vi "viewerMain.vi"(1 "viewer.lvclass":refnum<class "viewer.lvclass">) -> (0 "viewer.lvclass 2":refnum<class "viewer.lvclass">)   [LabVIEW 2011, in "viewer.lvclass"]
uses:
  Pollers/ttm_poller_panel_class/viewer.lvclass
  viewerDataVectors.ctl
  protocols/protocol_Generic/Protocol_Generic.lvclass
  viewerSingleGraph.ctl
panel:
  out "protocol Runner error":errorcluster
  in  "ttmServer vi":path=path "D:/workspace/lumikki-devices/ttm/protocols/run_protocols/main.vi"
  in  "Updade frequency [ms]":u32=1000
  in  "Scales":T1={"Scale time"=1.0, "Scale analog displacement"=1.0, "Scale force"=1.0, "Scale digital displacement"=1.0, "Scale external"=1.0}
  in  "Tab Control":T2(tab)=enum."Force-displacement"
  in  "Front panel name":u16(ring) items=["select front panel", "Run_protocols.lvclass:main.vi"]
  out "Force-displacement":cluster{"Y":dbl[], "Y":dbl[]}[](graph)=[{"Y"=[0.5311861979208834, 0.5311861979208834, 0.6668696350036979, 0.7379313711099627, 0.8016199408837772, 0.8572989891886034, 0.9044121893788258, 0.9424888019316975, 0.9711483779210446, 0.9901045603371778, 0.999167945271476, 0.9982479743776325, 0.9873538397007164, 0.9665943918332975, 0.9361770523163061, 0.89640574115156, 0.8476778401335698, 0.7904802223420048, 0.7253843874668195, 0.6530407515722648, 0.5741721483545726, 0.4895666068265995, 0.4000694775924195, 0.30657498638352293, 0.21001729925089915, 0.11136118868665001, 0.011592393936158275, -0.0882922281826076, -0.18729466354290317, -0.28442571253646254, -0.3787148738289976], "Y"=[0.36472117505578305, 0.36472117505578305, 0.46768216950310704, 0.5255260682597803, 0.5810351605373051, 0.6339628306183481, 0.684073931524491, 0.7311458297268958, 0.7749693942622354, 0.8153499258594433, 0.852108021949363, 0.8850803737142298, 0.9141204916358583, 0.9390993563190676, 0.9599059916988695, 0.9764479580847747, 0.9886517628517197, 0.9964631869529988, 0.9998475258045683, 0.998789743470524, 0.9932945394647364, 0.9833863278718569, 0.9691091288804563, 0.9505263732101938, 0.9277206203019036, 0.9007931915226273, 0.8698637200151869, 0.8350696191922243, 0.7965654722360865, 0.7545223453168781, 0.7091270275799205]}]
  out "X-time":cluster{"Y":dbl[], "Y":dbl[]}[](graph)=[{"Y"=[56.0, 56.0, 73.0, 83.0, 93.0, 103.0, 113.0, 123.0, 133.0, 143.0, 153.0, 163.0, 173.0, 183.0, 193.0, 203.0, 213.0, 223.0, 233.0, 243.0, 253.0, 263.0, 273.0, 283.0, 293.0, 303.0, 313.0, 323.0, 333.0, 343.0, 353.0], "Y"=[0.5311861979208834, 0.5311861979208834, 0.6668696350036979, 0.7379313711099627, 0.8016199408837772, 0.8572989891886034, 0.9044121893788258, 0.9424888019316975, 0.9711483779210446, 0.9901045603371778, 0.999167945271476, 0.9982479743776325, 0.9873538397007164, 0.9665943918332975, 0.9361770523163061, 0.89640574115156, 0.8476778401335698, 0.7904802223420048, 0.7253843874668195, 0.6530407515722648, 0.5741721483545726, 0.4895666068265995, 0.4000694775924195, 0.30657498638352293, 0.21001729925089915, 0.11136118868665001, 0.011592393936158275, -0.0882922281826076, -0.18729466354290317, -0.28442571253646254, -0.3787148738289976]}, {"Y"=[56.0, 56.0, 73.0, 83.0, 93.0, 103.0, 113.0, 123.0, 133.0, 143.0, 153.0, 163.0, 173.0, 183.0, 193.0, 203.0, 213.0, 223.0, 233.0, 243.0, 253.0, 263.0, 273.0, 283.0, 293.0, 303.0, 313.0, 323.0, 333.0, 343.0, 353.0], "Y"=[0.36472117505578305, 0.36472117505578305, 0.46768216950310704, 0.5255260682597803, 0.5810351605373051, 0.6339628306183481, 0.684073931524491, 0.7311458297268958, 0.7749693942622354, 0.8153499258594433, 0.852108021949363, 0.8850803737142298, 0.9141204916358583, 0.9390993563190676, 0.9599059916988695, 0.9764479580847747, 0.9886517628517197, 0.9964631869529988, 0.9998475258045683, 0.998789743470524, 0.9932945394647364, 0.9833863278718569, 0.9691091288804563, 0.9505263732101938, 0.9277206203019036, 0.9007931915226273, 0.8698637200151869, 0.8350696191922243, 0.7965654722360865, 0.7545223453168781, 0.7091270275799205]}, {"Y"=[56.0, 56.0, 73.0, 83.0, 93.0, 103.0, 113.0, 123.0, 133.0, 143.0, 153.0, 163.0, 173.0, 183.0, 193.0, 203.0, 213.0, 223.0, 233.0, 243.0, 253.0, 263.0, 273.0, 283.0, 293.0, 303.0, 313.0, 323.0, 333.0, 343.0, 353.0], "Y"=[0.27635564856411376, 0.27635564856411376, 0.35694929447691137, 0.4031899303856266, 0.44842280144563446, 0.49253484903610867, 0.5354158160111833, 0.5769585222853968, 0.6170591327280867, 0.6556174166971402, 0.6925369985634013, 0.7277255985995504, 0.7610952636313663, 0.7925625868748546, 0.8220489164097717, 0.8494805517684643, 0.8747889281486548, 0.8979107877897406, 0.9187883380842506, 0.9373693960292665, 0.9536075186567536, 0.9674621191167943, 0.9788985681235746, 0.9878882805105652, 0.9944087866785504, 0.998443788757924, 0.9999832013448761, 0.9990231767096499, 0.9955661144138624, 0.9896206553128498, 0.9812016599580293]}, {"Y"=[56.0, 56.0, 73.0, 83.0, 93.0, 103.0, 113.0, 123.0, 133.0, 143.0, 153.0, 163.0, 173.0, 183.0, 193.0, 203.0, 213.0, 223.0, 233.0, 243.0, 253.0, 263.0, 273.0, 283.0, 293.0, 303.0, 313.0, 323.0, 333.0, 343.0, 353.0], "Y"=[0.2221314566339704, 0.2221314566339704, 0.2878681396739431, 0.3259344637346948, 0.3634793621824483, 0.4004427711888383, 0.43676555718456145, 0.4723896114604721, 0.5072579431291219, 0.5413147702980217, 0.5745056093087701, 0.6067773618992848, 0.6380784001496942, 0.6683586490759965, 0.6975696667393515, 0.7256647217428491, 0.7525988679917759, 0.7783290165977784, 0.8028140048118926, 0.8260146618761615, 0.8478938716884917, 0.8684166321804996, 0.887550111313353, 0.9052636996020308, 0.9215290590839683, 0.9363201686537528, 0.9496133656913409, 0.9613873839172035, 0.9716233874138356, 0.9803050007592069, 0.9874183352239436]}]
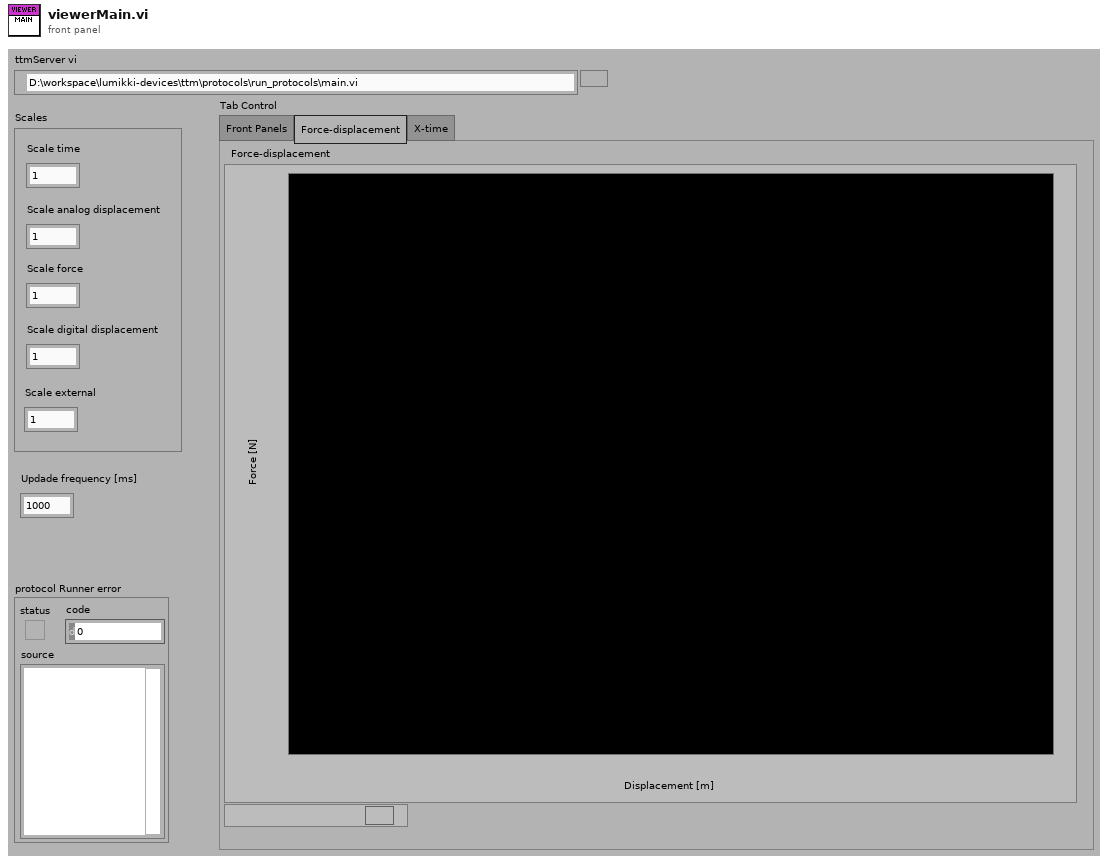
[diagram p1: front panel]
types:
  T1 = cluster{"Scale time":dbl, "Scale analog displacement":dbl, "Scale force":dbl, "Scale digital displacement":dbl, "Scale external":dbl}
  T2 = enum32{"Front Panels", "Force-displacement", "X-time"}
  T3 = typedef "viewer.lvclass/viewerDataVectors.ctl" = cluster{"time":dbl[], "analogDisplacement":dbl[], "external":dbl[], "force":dbl[], "digitalDisplacement":dbl[]}
  T4 = typedef "viewer.lvclass/viewerSingleGraph.ctl" = cluster{"X":dbl[], "Y":dbl[]}
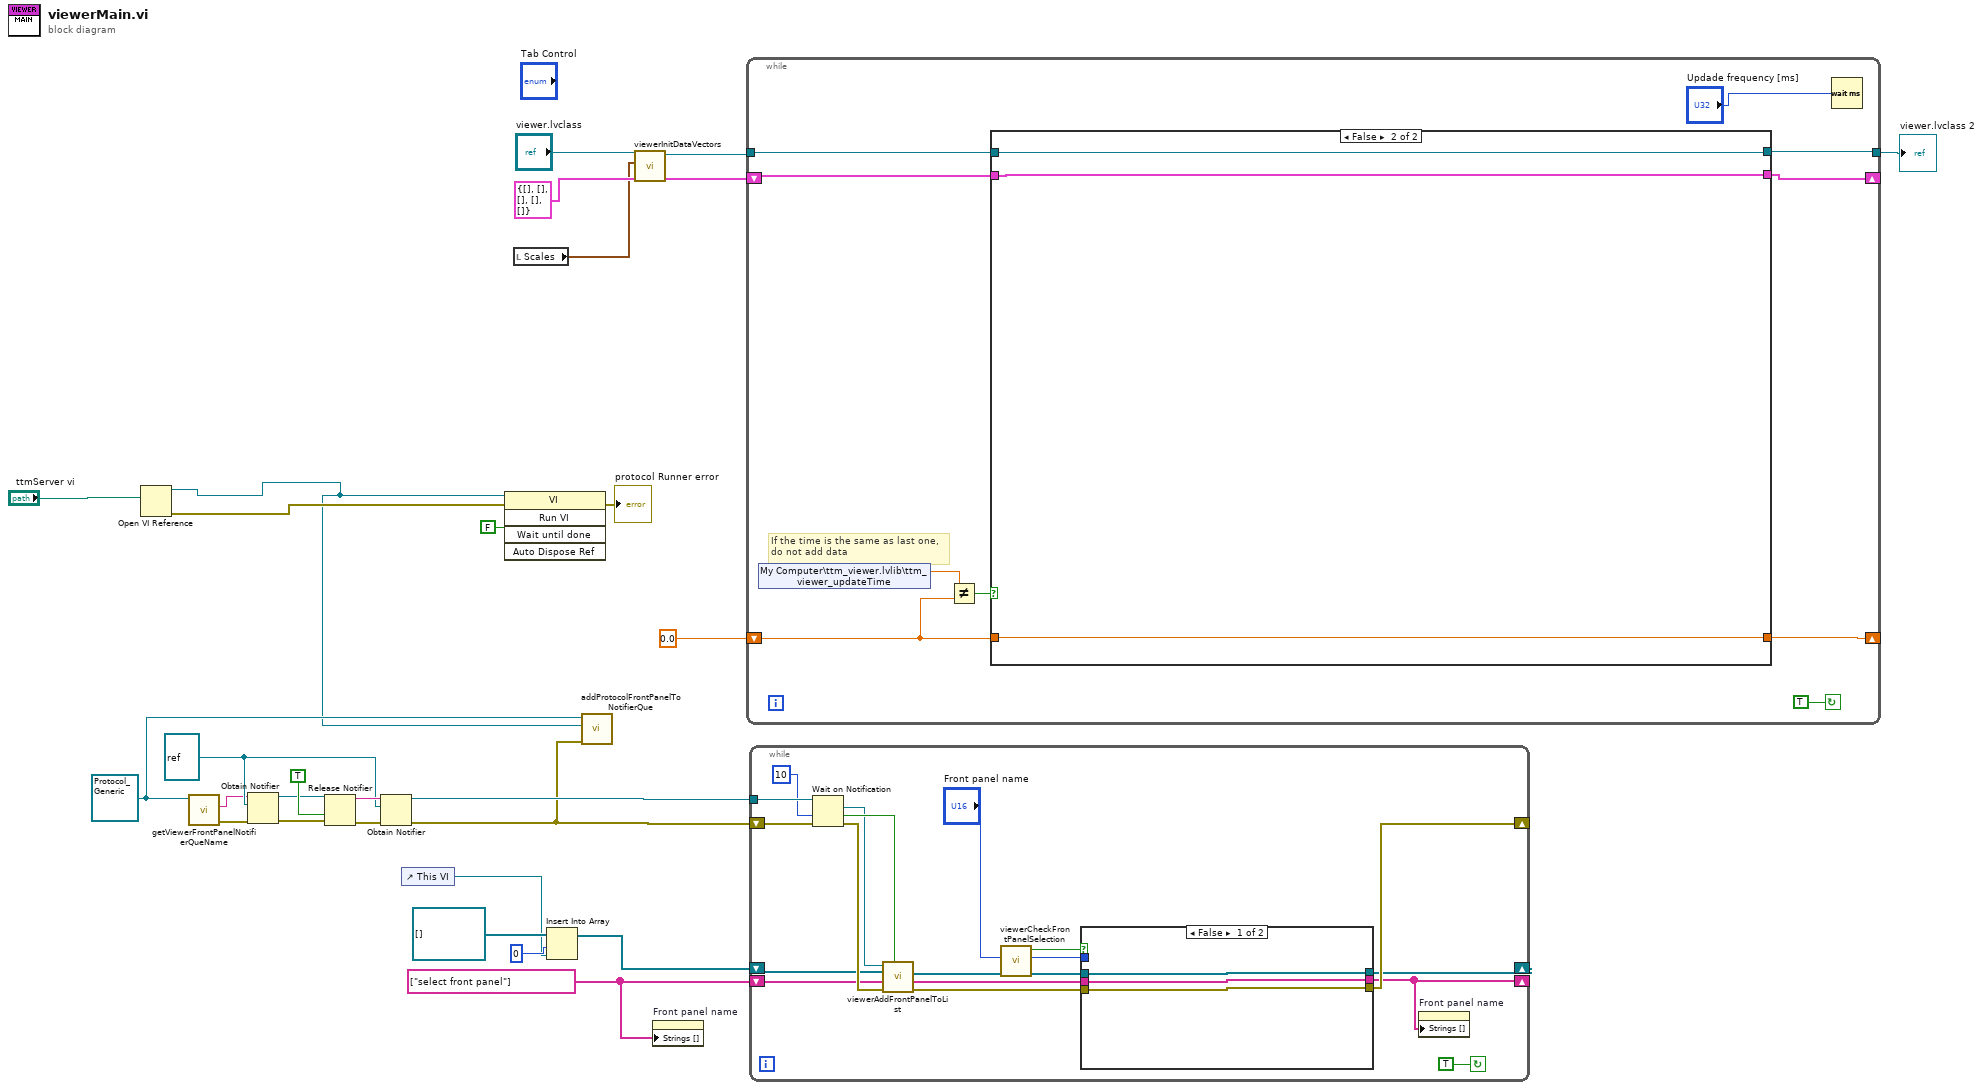
[diagram p0: block diagram]
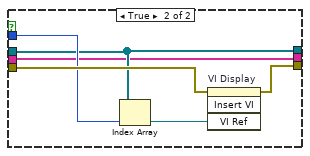
[diagram p2: hidden frame]
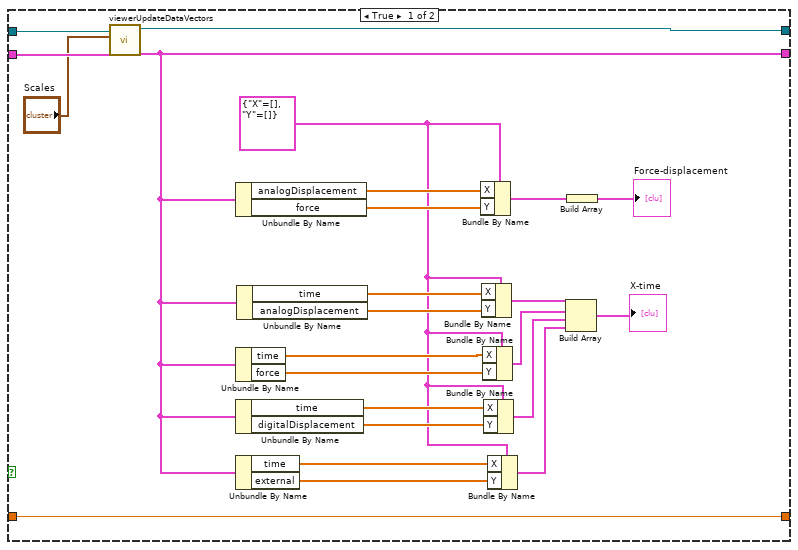
[diagram p3: hidden frame]
diagram:
  w6 = refnum<class "Protocol_Generic.lvclass"> refnum ("Protocol_Generic.lvclass")
  w14 = string[] ["select front panel"]
  w15 = refnum<vi> refnum ("protocolFrontPanel")
  n1 = Open VI Reference(vi path="ttmServer vi") -> (vi reference=w2:refnum<vi>, error out=w5:errorcluster)  [unwired: 5 in]
  n2 = call-dynamic "getViewerFrontPanelNotifierQueName.vi"("Protocol_Generic in"=w6) -> ("error out"=w12:errorcluster, "viewerFrontPanelNotifierQueName"=w13:string)  [unwired: 8 in, 1 out]
  n3 = Obtain Notifier(name (unnamed)=w13, notification data type=w15, error in (no error)=w12) -> (notifier out=w19:refnum<notifier>, error out=w20:errorcluster)  [unwired: 1 in, 1 out]
  n4 = Release Notifier(notifier=w19, force destroy? (F)=TRUE, error in (no error)=w20) -> (notifier name=w18:string, error out=w17:errorcluster)  [unwired: 1 out]
  n5 = Obtain Notifier(name (unnamed)=w18, notification data type=w15, error in (no error)=w17) -> (notifier out=w16:refnum<notifier>, error out=w7:errorcluster)  [unwired: 1 in, 1 out]
  n6 = control-ref of="This VI"() -> (w8:refnum<vi>)
  n7 = invoke class="VI" method="Run VI"(reference=w2, error in=w5, "Wait until done"=FALSE) -> (error out=→"protocol Runner error":errorcluster)  [unwired: 2 in, 4 out]
  n8 = local read "Scales"() -> (w22:T1)
  n9 = Insert Into Array(array=refnum<vi>[] [], index=0, new element=w8) -> (w9:refnum<vi>[])
  n10 = call-dynamic "addProtocolFrontPanelToNotifierQue.vi"("error in (no error)"=w7, "frontPanelReference"=w2, "Protocol_Generic in"=w6) -> ()  [unwired: 7 in, 2 out]
  n11 = call "viewerInitDataVectors.vi"("viewerDataVectors"=T3 {"time"=[], "analogDisplacement"=[], "external"=[], "force"=[], "digitalDisplacement"=[]}, "Cluster"=w22, "viewer.lvclass"="viewer.lvclass") -> ("viewerDataVectorsOut"=w23:T3, "viewer.lvclassOut"=w24:refnum<class "viewer.lvclass">)  [unwired: 7 in]
  n12 = property on="Front panel name" class="Ring (strict)"("Strings []"=w14) -> ()  [unwired: 2 in, 2 out]
  n13 = while {
    shift-right: [w37] -> _
    shift-left: 0.0 ("Double") -> [w32]
    shift-right: [w33] -> _
    shift-left: w23 -> [w34]
    tunnel: w24 -> [w36]
    tunnel: [w35] -> w27
    stop <- TRUE continue-if-true
    # "If the time is the same as last one,\ndo not add data"
    n14 = shared-variable "My Computer\\ttm_viewer.lvlib\\ttm_viewer_updateTime"() -> (w31:dbl)  [unwired: 1 in, 1 out]
    n15 = Not Equal?(x=w31, y=w32) -> (x != y?=w38:bool)
    n16 = case shown="False" w38 {
      tunnel: w32 -> [w50 w64]
      tunnel: [w50 w64] -> w37
      tunnel: w36 -> [w58 w65]
      tunnel: [w41 w65] -> w35
      tunnel: w34 -> [w57 w63]
      tunnel: [w46 w63] -> w33
      frame True {
        w40 = T4 {"X"=[], "Y"=[]} ("Graph")
        n17 = call "viewerUpdateDataVectors.vi"("viewerDataVectors"=w57, "Cluster"="Scales", "viewer.lvclass"=w58) -> ("viewerDataVectorsOut"=w46:T3, "viewer.lvclassOut"=w41:refnum<class "viewer.lvclass">)  [unwired: 7 in]
        n18 = Unbundle By Name(w46) -> ("analogDisplacement"=w61:dbl[], "force"=w62:dbl[])
        n19 = Unbundle By Name(w46) -> ("time"=w54:dbl[], "force"=w53:dbl[])
        n20 = Unbundle By Name(w46) -> ("time"=w49:dbl[], "digitalDisplacement"=w48:dbl[])
        n21 = Unbundle By Name(w46) -> ("time"=w45:dbl[], "external"=w44:dbl[])
        n22 = Unbundle By Name(w46) -> ("time"=w56:dbl[], "analogDisplacement"=w55:dbl[])
        n23 = Bundle By Name(cluster=w40, "X"=w61, "Y"=w62) -> (w60:T4)
        n24 = Bundle By Name(cluster=w40, "X"=w56, "Y"=w55) -> (w52:T4)
        n25 = Bundle By Name(cluster=w40, "X"=w54, "Y"=w53) -> (w51:T4)
        n26 = Bundle By Name(cluster=w40, "X"=w49, "Y"=w48) -> (w47:T4)
        n27 = Bundle By Name(cluster=w40, "X"=w45, "Y"=w44) -> (w43:T4)
        n28 = Build Array(w52, w51, w47, w43) -> (→"X-time":T4[])
        n29 = Build Array(w60) -> (→"Force-displacement":T4[])
      }
      frame False {
      }
    }
    n30 = Wait (ms)(milliseconds to wait="Updade frequency [ms]") -> ()  [unwired: 1 out]
  }
  "viewer.lvclass 2" <- w27
  n31 = while {
    tunnel: w16 -> [w83]
    shift-right: [w77] -> _
    shift-left: w9 -> [w74]
    shift-right: [w76] -> _
    shift-left: w14 -> [w73]
    shift-right: [w79] -> _
    shift-left: w7 -> [w75]
    stop <- TRUE continue-if-true
    n32 = Wait on Notification(notifier=w83, timeout in ms (-1)=10, error in (no error)=w75) -> (notification=w78:refnum<vi>, timed out?=w82:bool, error out=w80:errorcluster)  [unwired: 1 in, 1 out]
    n33 = call "viewerAddFrontPanelToList.vi"("NoNewPanels?"=w82, "error in (no error)"=w80, "selectorNameListIn"=w73, "selectorReferenceListIn"=w74, "viReferenceIn"=w78) -> ("error out"=w72:errorcluster, "selectorNameListOut"=w71:string[], "selectorReferenceListOut"=w68:refnum<vi>[])  [unwired: 3 in, 1 out]
    n34 = call "viewerCheckFrontPanelSelection.vi"("selectorReferenceListIn"=w68, "frontPanelIndexIn"="Front panel name") -> ("selectorReferenceListOut"=w67:refnum<vi>[], "frontPanelIndexOut"=w69:u16, "ShowFrontPanel"=w66:bool)  [unwired: 7 in]
    n35 = case shown="False" w66 {
      tunnel: w67 -> [w86 w89]
      tunnel: w72 -> [w87 w92]
      tunnel: [w87 w91] -> w79
      tunnel: w69 -> [_ w90]
      tunnel: [w86 w89] -> w77
      tunnel: w71 -> [w85 w88]
      tunnel: [w85 w88] -> w76
      frame False {
      }
      frame True {
        n36 = Index Array(array=w89, index=w90) -> (element=w93:refnum<vi>)
        n37 = invoke on="VI Display" class="SubPnl" method="Insert VI"(error in=w92, "VI Ref"=w93) -> (error out=w91:errorcluster)  [unwired: 2 in, 3 out]
      }
    }
    n38 = property on="Front panel name" class="Ring (strict)"("Strings []"=w76) -> ()  [unwired: 2 in, 2 out]
  }
